vi "Begin.vi"() -> (0 "CameraDevRef 2":T1, 1 "CameraDevRef":T1)   [LabVIEW 2011]
doc: "Called before other user functions, this VI is expected to open initial I/O refnums, load in file data, and do all program initialization. Notice that the <B>error out</B> terminal is simply used for data flow. Wiring it to other structures or subVIs ensures that this VI runs first."
uses:
  <vilib>/Rock Robotics/WPI/Camera/WPI_CameraDevRef.ctl
  <vilib>/Rock Robotics/SystemInterfaces/DIO/FPGA_DIOPWMChannel.ctl
  <vilib>/Rock Robotics/WPI/Joystick/WPI_JoystickDeviceEnum.ctl
  <vilib>/Rock Robotics/SystemInterfaces/AI/FPGA_AIChannel.ctl
  <vilib>/Rock Robotics/SystemInterfaces/DIO/FPGA_DIORelayChannel.ctl
  <vilib>/Rock Robotics/SystemInterfaces/DIO/FPGA_DIOChannel.ctl
  <vilib>/Rock Robotics/SystemInterfaces/AI/FPGA_AIGyroChannel.ctl
  <vilib>/Rock Robotics/WPI/Relay/WPI_RelayDirection.ctl
  <vilib>/Rock Robotics/WPI/Encoder/WPI_EncoderType.ctl
  <vilib>/Rock Robotics/WPI/DriverStation/DriverStationLCD/WPI_DriverStationLCDLCDLine.ctl
  <vilib>/Rock Robotics/WPI/MotorControl/WPI_MotorControlOpen Victor.vi
  <vilib>/Rock Robotics/WPI/MotorControl/WPI_MotorControlOpen Jaguar.vi
  Robot Global Data.vi
  <vilib>/Utility/file.llb/Read From Spreadsheet File (DBL).vi
  <vilib>/Rock Robotics/WPI/Counter/WPI_CounterDigitalInputToDigitalSource.vi
  <vilib>/Rock Robotics/SystemInterfaces/Typedef/FPGA_TypedefDigitalModule.ctl
  <vilib>/Rock Robotics/SystemInterfaces/Typedef/FPGA_TypedefAnalogModule.ctl
panel:
  in  "Default Shooter in Feet":i32=13
  out "Path and file":string
  in  "Balls In Robot At Start":dbl=2.0
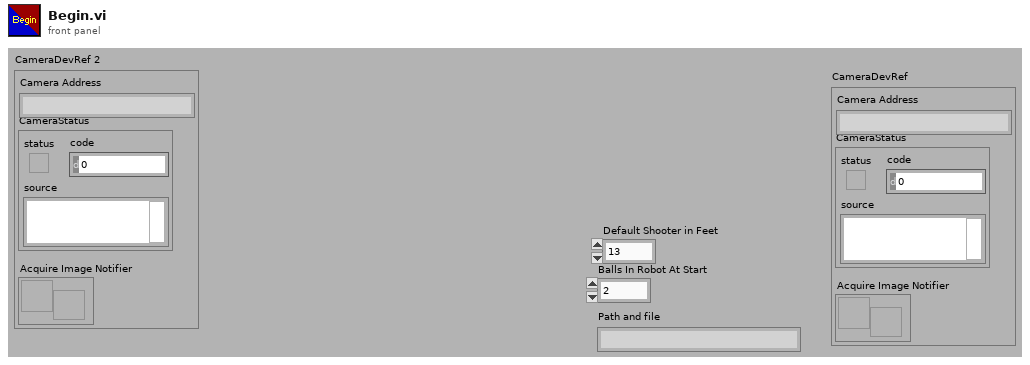
[diagram p1: front panel]
types:
  T1 = typedef "WPI_CameraDevRef.ctl" = cluster{"Camera Address":string, "CameraStatus":errorcluster, "Acquire Image Notifier":refnum<notifier>}
  T2 = typedef "FPGA_DIOChannel.ctl" = enum8{"DIO 1", "DIO 2", "DIO 3", "DIO 4", "DIO 5", "DIO 6", "DIO 7", "DIO 8", "DIO 9", "DIO 10", "DIO 11", "DIO 12", "DIO 13", "DIO 14", "Invalid"}
  T3 = typedef "FPGA_DIOPWMChannel.ctl" = enum8{"PWM 1", "PWM 2", "PWM 3", "PWM 4", "PWM 5", "PWM 6", "PWM 7", "PWM 8", "PWM 9", "PWM 10", "Invalid"}
  T4 = typedef "WPI_DriverStationLCDLCDLine.ctl" = enum16{"Main - Line 1", "User - Line 2", "User - Line 3", "User - Line 4", "User - Line 5", "User - Line 6"}
  T5 = typedef "WPI_EncoderType.ctl" = enum16{"1x", "2x", "4x"}
  T6 = typedef "FPGA_DIORelayChannel.ctl" = enum8{"Relay 1", "Relay 2", "Relay 3", "Relay 4", "Relay 5", "Relay 6", "Relay 7", "Relay 8", "Invalid"}
  T7 = typedef "WPI_RelayDirection.ctl" = enum16{"Both directions", "Forward only", "Reverse only"}
  T8 = typedef "FPGA_AIGyroChannel.ctl" = enum8{"AI 1", "AI 2", "Invalid"}
  T9 = typedef "FPGA_AIChannel.ctl" = enum8{"AI 1", "AI 2", "AI 3", "AI 4", "AI 5", "AI 6", "AI 7", "AI 8", "Invalid"}
  T10 = typedef "WPI_JoystickDeviceEnum.ctl" = enum16{"USB 1", "USB 2", "USB 3", "USB 4", "Kinect 1", "Kinect 2"}
  T11 = typedef "WPI_CameraImageSize.ctl" = enum16{"640x480", "320x240", "160x120"}
  T12 = cluster{"fps":i32, "compression":i32, "Image Size":T11}
  T13 = typedef "WPI_MotorControlDeviceRef.ctl" = cluster{"DeviceStatus":errorcluster, "Type":enum16{"PWM", "CAN"}, "PWM":cluster{"Digital Module":T14, "PWM Channel":T3, "DeadBand":T15}, "CAN":cluster{"Device Number":u8, "Control Mode":T16, "Semaphore":T17, "Max Vout":dbl}, "Invert":bool, "TransformRef":T18, "InvTransformRef":T18}
  T14 = typedef "FPGA_TypedefDigitalModule.ctl" = enum16{"Digital Module 1", "Digital Module 2"}
  T15 = typedef "WPI_PWMDeadband.ctl" = cluster{"Name":string, "maxPositivePwm":i32, "minPositivePwm":i32, "centerPwm":i32, "maxNegativePwm":i32, "minNegativePwm":i32, "angularRange":u16}
  T16 = typedef "WPI_CANJaguar_ControlMode.ctl" = enum8{"Percent VBus", "Current", "Speed", "Position", "Voltage"}
  T17 = typedef "Semaphore RefNum" = refnum<k1>
  T18 = typedef "WPI_PWMTransform_ConPane.ctl" = refnum<vi>
  T19 = typedef "WPI_ServoDeviceRef.ctl" = cluster{"DeviceStatus":errorcluster, "Digital Module":T14, "PWM Channel":T3, "DeadBand":T15}
  T20 = typedef "WPI_AnalogChannelDevRef.ctl" = cluster{"DevStatus":errorcluster, "Analog Module":T21, "Analog Channel":T9}
  T21 = typedef "FPGA_TypedefAnalogModule.ctl" = enum16{"Analog Module 1", "Analog Module 2"}
  T22 = typedef "WPI_CameraWhite Balance Values.ctl" = enum16{"Auto", "Fixed indoor", "Fixed outdoor 1", "Fixed outdoor 2", "Fixed fluorescent 1", "Fixed fluorescent 2", "Hold current"}
  T23 = typedef "WPI_JoystickDevRef.ctl" = cluster{"Device":T10}
  T24 = typedef "WPI_RelayDevRef.ctl" = cluster{"DevStatus":errorcluster, "Relay Channel":T6, "Digital Module":T14, "Relay Direction":T7}
  T25 = typedef "WPI_CameraExposure Values.ctl" = enum16{"Auto", "Flicker-free 50 Hz", "Flicker-free 60 Hz", "Hold current"}
  T26 = typedef "WPI_DigitalInputDevRef.ctl" = cluster{"DevStatus":errorcluster, "DIO Channel":T2, "Digital Module":T14}
  T27 = typedef "FPGA_CounterEncoderSourceConvertionLVSourceType.ctl" = cluster{"DevStatus":errorcluster, "AnalogTriggerMode?":bool, "DigitalMode":cluster{"Digital Module":T14, "DIO Channel":T28}, "AnalogTriggerMode":cluster{"AnalogTriggerIndex":T29, "OutputType":T30}}
  T28 = typedef "FPGA_DIODigitalSourceChannel.ctl" = enum8{"DIO 1", "DIO 2", "DIO 3", "DIO 4", "DIO 5", "DIO 6", "DIO 7", "DIO 8", "DIO 9", "DIO 10", "DIO 11", "DIO 12", "DIO 13", "DIO 14", "Disabled"}
  T29 = typedef "FPGA_AnalogTriggerIndex.ctl" = enum8{"Trig 0", "Trig 1", "Trig 2", "Trig 3", "Trig 4", "Trig 5", "Trig 6", "Trig 7", "Invalid"}
  T30 = typedef "FPGA_AnalogTriggerOutType.ctl" = enum16{"InWindow", "TriggerState", "Rising", "Falling"}
  T31 = typedef "WPI_EncoderDevRef.ctl" = cluster{"DevStatus":errorcluster, "EncoderIndex":T32, "CounterIndex":T33, "DistancePerCount":dbl, "Decoding Type":T5}
  T32 = typedef "FPGA_EncoderIdx.ctl" = enum8{"Enc 0", "Enc 1", "Enc 2", "Enc 3", "Invalid"}
  T33 = typedef "FPGA_CounterCtrSystemIndex.ctl" = enum8{"Ctr 0", "Ctr 1", "Ctr 2", "Ctr 3", "Ctr 4", "Ctr 5", "Ctr 6", "Ctr 7", "Invalid"}
  T34 = typedef "WPI_GyroDevRef.ctl" = cluster{"DevStatus":errorcluster, "Analog Module":T21, "Analog Channel":T9, "Offset":dbl, "Gain (VoltsPerDegree/Second)":dbl}
  T35 = typedef "WPI_UltrasonicDeviceRef.ctl" = cluster{"DevStatus":errorcluster, "Ping Digital Module":T14, "Echo Digital Module":T14, "Ping Channel":T2, "Echo Channel":T2, "CntIndex":T33}
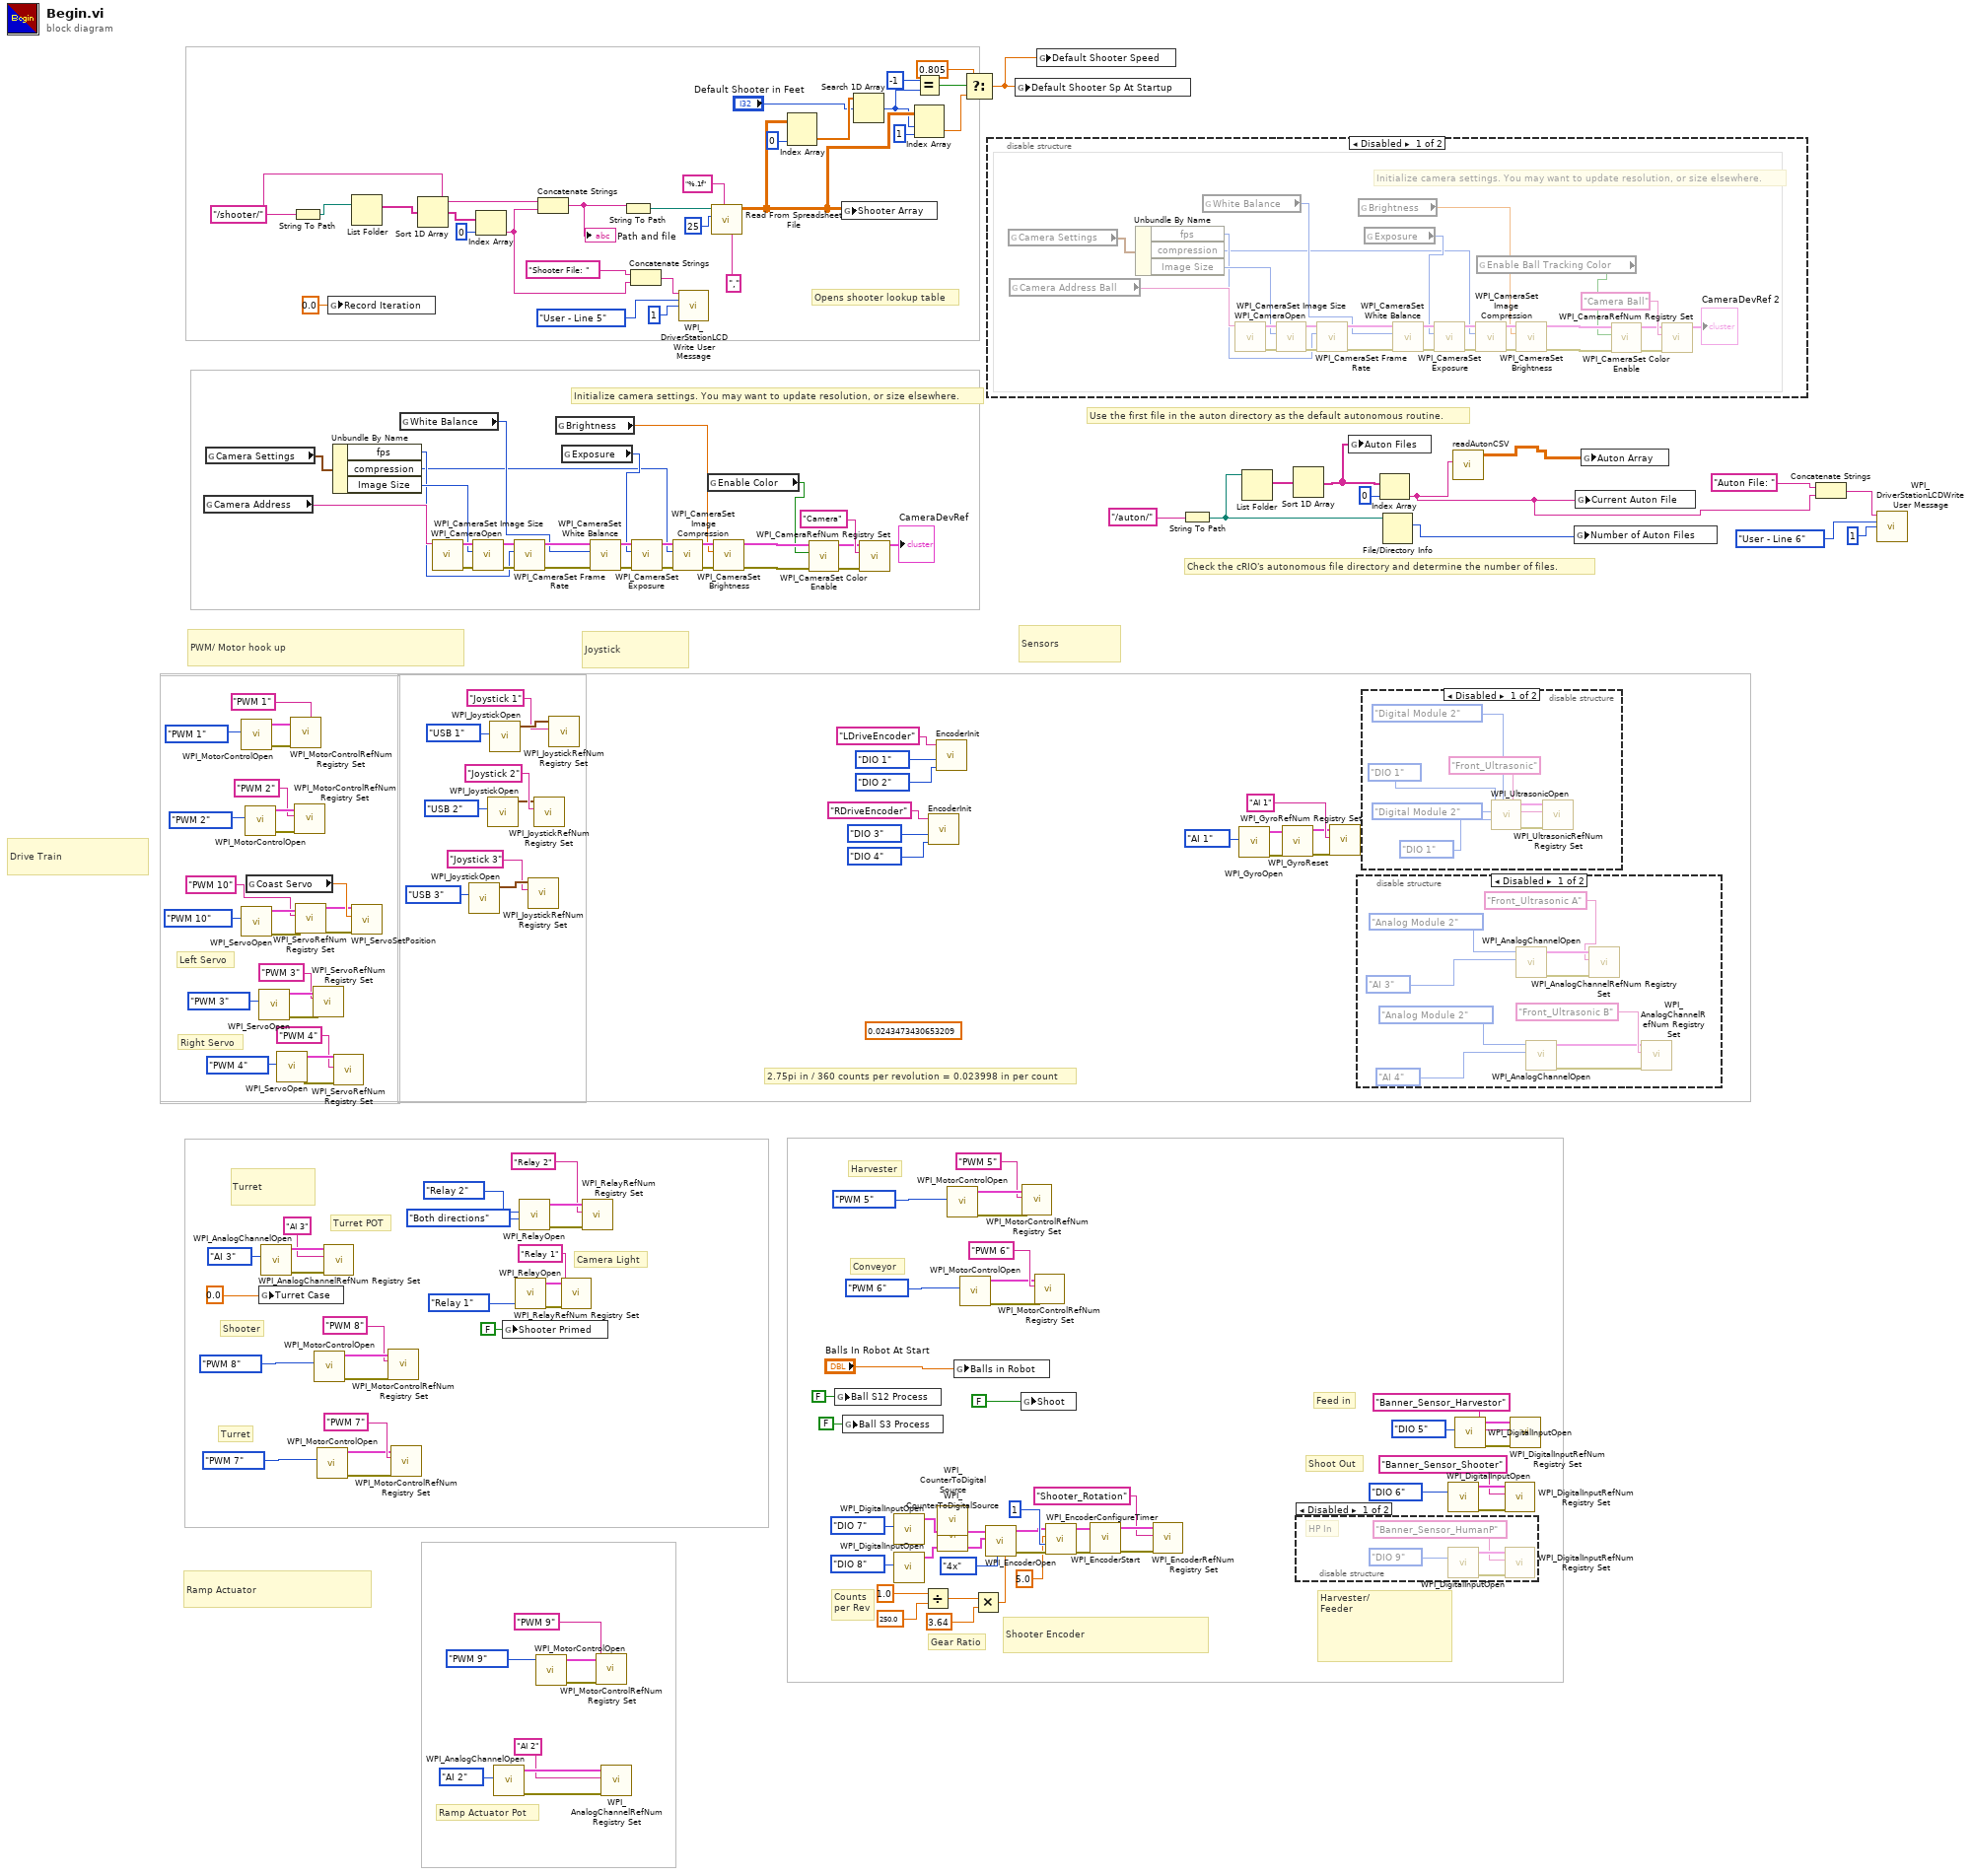
[diagram p0: block diagram]
diagram:
  (unwired) 0.0243473430653209 ("DistancePerCount")
  w70 = "/shooter/" ("string")
  # "Shooter Encoder"
  # "Counts\nper Rev"
  # "Gear Ratio"
  # "Check the cRIO's autonomous file directory and determine the number of files."
  # "Use the first file in the auton directory as the default autonomous routine."
  # "2.75pi in / 360 counts per revolution = 0.023998 in per count"
  # "Opens shooter lookup table"
  # "Shoot Out"
  # "Feed in"
  # "Harvester"
  # "Conveyor"
  # "Shooter"
  # "Initialize camera settings. You may want to update resolution, or size elsewhere."
  # "Camera Light"
  # "Ramp Actuator Pot"
  # "Turret POT"
  # "Turret"
  # "Right Servo"
  # "Left Servo"
  # "Harvester/\nFeeder"
  # "Turret"
  # "Ramp Actuator"
  # "Drive Train"
  # "Sensors"
  # "Joystick"
  # "PWM/ Motor hook up"
  n1 = global read "Robot Global Data.vi" "Camera Address"() -> (w123:string)
  n2 = global read "Robot Global Data.vi" "Camera Settings"() -> (w122:T12)
  n3 = call-poly <vilib>:"WPI_MotorControlOpen.vi"("PWM Channel"=FPGA_DIOPWMChannel."PWM 1") -> ("error out"=w163:errorcluster, "MotorControlDeviceRef"=w165:T13)  [unwired: 9 in]
  n4 = call <vilib>:"WPI_ServoOpen.vi"("PWM Channel"=FPGA_DIOPWMChannel."PWM 10") -> ("error out"=w19:errorcluster, "ServoDeviceRef"=w23:T19)  [unwired: 9 in]
  n5 = call-poly <vilib>:"WPI_MotorControlOpen.vi"("PWM Channel"=FPGA_DIOPWMChannel."PWM 2") -> ("error out"=w161:errorcluster, "MotorControlDeviceRef"=w159:T13)  [unwired: 9 in]
  n6 = global read "Robot Global Data.vi" "Coast Servo"() -> (w24:dbl)
  n7 = call <vilib>:"WPI_ServoOpen.vi"("PWM Channel"=FPGA_DIOPWMChannel."PWM 3") -> ("error out"=w176:errorcluster, "ServoDeviceRef"=w181:T19)  [unwired: 9 in]
  n8 = global write "Robot Global Data.vi" "Turret Case"(0.0 ("Return To Home Case")) -> ()
  n9 = call <vilib>:"WPI_AnalogChannelOpen.vi"("Analog Channel"=FPGA_AIChannel."AI 3") -> ("error out"=w152:errorcluster, "AIDeviceRef"=w153:T20)  [unwired: 9 in]
  n10 = call <vilib>:"WPI_ServoOpen.vi"("PWM Channel"=FPGA_DIOPWMChannel."PWM 4") -> ("error out"=w175:errorcluster, "ServoDeviceRef"=w179:T19)  [unwired: 9 in]
  n11 = call <vilib>:"WPI_MotorControlRefNum Registry Set.vi"("error in (no error)"=w163, "refnum name"="PWM 1", "MotorControlDevRef"=w165) -> ()  [unwired: 7 in, 2 out]
  n12 = String To Path(string=w70) -> (path=w79:path)
  n13 = call <vilib>:"WPI_MotorControlRefNum Registry Set.vi"("error in (no error)"=w161, "refnum name"="PWM 2", "MotorControlDevRef"=w159) -> ()  [unwired: 7 in, 2 out]
  n14 = call <vilib>:"WPI_ServoRefNum Registry Set.vi"("error in (no error)"=w19, "refnum name"="PWM 10", "ServoDeviceRef"=w23) -> ("error out"=w20:errorcluster, "ServoDeviceRef"=w21:T19)  [unwired: 7 in]
  n15 = call <vilib>:"WPI_ServoRefNum Registry Set.vi"("error in (no error)"=w176, "refnum name"="PWM 3", "ServoDeviceRef"=w181) -> ()  [unwired: 7 in, 2 out]
  n16 = call-poly <vilib>:"WPI_MotorControlOpen.vi"("PWM Channel"=FPGA_DIOPWMChannel."PWM 8") -> ("error out"=w106:errorcluster, "MotorControlDeviceRef"=w108:T13)  [unwired: 9 in]
  n17 = call-poly <vilib>:"WPI_MotorControlOpen.vi"("PWM Channel"=FPGA_DIOPWMChannel."PWM 7") -> ("error out"=w157:errorcluster, "MotorControlDeviceRef"=w155:T13)  [unwired: 9 in]
  n18 = call <vilib>:"WPI_AnalogChannelRefNum Registry Set.vi"("error in (no error)"=w152, "refnum name"="AI 3", "AIDeviceRef"=w153) -> ()  [unwired: 7 in, 2 out]
  n19 = global write "Robot Global Data.vi" "Record Iteration"(0.0 ("Record Iteration")) -> ()
  n20 = Unbundle By Name(w122) -> ("fps"=w120:i32, "compression"=w117:i32, "Image Size"=w121:T11)
  n21 = call <vilib>:"WPI_ServoRefNum Registry Set.vi"("error in (no error)"=w175, "refnum name"="PWM 4", "ServoDeviceRef"=w179) -> ()  [unwired: 7 in, 2 out]
  n22 = List Folder(path=w79) -> (filenames=w78:string[])  [unwired: 1 in, 5 out]
  n23 = call <vilib>:"WPI_ServoSetPosition.vi"("error in (no error)"=w20, "Position"=w24, "ServoDeviceRef"=w21) -> ()  [unwired: 7 in, 2 out]
  n24 = call <vilib>:"WPI_MotorControlRefNum Registry Set.vi"("error in (no error)"=w106, "refnum name"="PWM 8", "MotorControlDevRef"=w108) -> ()  [unwired: 7 in, 2 out]
  n25 = call <vilib>:"WPI_MotorControlRefNum Registry Set.vi"("error in (no error)"=w157, "refnum name"="PWM 7", "MotorControlDevRef"=w155) -> ()  [unwired: 7 in, 2 out]
  n26 = global read "Robot Global Data.vi" "White Balance"() -> (w119:T22)
  n27 = Sort 1D Array(array=w78) -> (sorted array=w77:string[])
  n28 = call <vilib>:"WPI_CameraOpen.vi"("Camera Address"=w123) -> ("error out"=w129:errorcluster, "CameraDevRef"=w130:T1)  [unwired: 1 in, 8 out]
  n29 = call <vilib>:"WPI_JoystickOpen.vi"("JoystickDevice"=WPI_JoystickDeviceEnum."USB 3") -> ("JoystickDevRef"=w168:T23)  [unwired: 10 in]
  n30 = call <vilib>:"WPI_CameraSet Image Size.vi"("error in (no error)"=w129, "Image Size"=w121, "CameraDevRef"=w130) -> ("error out"=w128:errorcluster, "CameraDevRef Out"=w131:T1)  [unwired: 7 out]
  n31 = Index Array(array=w77, index=0) -> (element=w30:string)
  n32 = call <vilib>:"WPI_JoystickOpen.vi"("JoystickDevice"=WPI_JoystickDeviceEnum."USB 2") -> ("JoystickDevRef"=w171:T23)  [unwired: 10 in]
  n33 = call <vilib>:"WPI_JoystickOpen.vi"("JoystickDevice"=WPI_JoystickDeviceEnum."USB 1") -> ("JoystickDevRef"=w174:T23)  [unwired: 10 in]
  n34 = call <vilib>:"WPI_AnalogChannelOpen.vi"("Analog Channel"=FPGA_AIChannel."AI 2") -> ("error out"=w147:errorcluster, "AIDeviceRef"=w148:T20)  [unwired: 9 in]
  n35 = global write "Robot Global Data.vi" "Shooter Primed"(FALSE ("Ball S3 Process")) -> ()
  n36 = call <vilib>:"WPI_CameraSet Frame Rate.vi"("error in (no error)"=w128, "Frame Rate (fps)"=w120, "CameraDevRef"=w131) -> ("error out"=w127:errorcluster, "CameraDevRef Out"=w133:T1)  [unwired: 7 out]
  n37 = call <vilib>:"WPI_RelayOpen.vi"("Relay Channel"=FPGA_DIORelayChannel."Relay 1") -> ("error out"=w140:errorcluster, "RelayDevRef"=w139:T24)  [unwired: 9 in]
  n38 = call <vilib>:"WPI_RelayOpen.vi"("Relay Direction"=WPI_RelayDirection."Both directions", "Relay Channel"=FPGA_DIORelayChannel."Relay 2") -> ("error out"=w66:errorcluster, "RelayDevRef"=w67:T24)  [unwired: 8 in]
  n39 = call <vilib>:"WPI_JoystickRefNum Registry Set.vi"("refnum name"="Joystick 3", "JoystickDevRef"=w168) -> ()  [unwired: 8 in, 2 out]
  n40 = call <vilib>:"WPI_JoystickRefNum Registry Set.vi"("refnum name"="Joystick 2", "JoystickDevRef"=w171) -> ()  [unwired: 8 in, 2 out]
  n41 = call-poly <vilib>:"WPI_MotorControlOpen.vi"("PWM Channel"=FPGA_DIOPWMChannel."PWM 9") -> ("error out"=w143:errorcluster, "MotorControlDeviceRef"=w144:T13)  [unwired: 9 in]
  n42 = Concatenate Strings(w70, w30) -> (w72:string)
  "Path and file" <- w72
  n43 = call <vilib>:"WPI_JoystickRefNum Registry Set.vi"("refnum name"="Joystick 1", "JoystickDevRef"=w174) -> ()  [unwired: 8 in, 2 out]
  n44 = global read "Robot Global Data.vi" "Brightness"() -> (w116:dbl)
  n45 = global read "Robot Global Data.vi" "Exposure"() -> (w118:T25)
  n46 = call <vilib>:"WPI_RelayRefNum Registry Set.vi"("error in (no error)"=w140, "refnum name"="Relay 1", "RelayDevRef"=w139) -> ()  [unwired: 7 in, 2 out]
  n47 = call <vilib>:"WPI_RelayRefNum Registry Set.vi"("error in (no error)"=w66, "refnum name"="Relay 2", "RelayDevRef"=w67) -> ()  [unwired: 7 in, 2 out]
  n48 = call <vilib>:"WPI_CameraSet White Balance.vi"("error in (no error)"=w127, "White Balance"=w119, "CameraDevRef"=w133) -> ("error out"=w126:errorcluster, "CameraDevRef Out"=w132:T1)  [unwired: 7 out]
  n49 = call <vilib>:"WPI_MotorControlRefNum Registry Set.vi"("error in (no error)"=w143, "refnum name"="PWM 9", "MotorControlDevRef"=w144) -> ()  [unwired: 7 in, 2 out]
  n50 = call <vilib>:"WPI_AnalogChannelRefNum Registry Set.vi"("error in (no error)"=w147, "refnum name"="AI 2", "AIDeviceRef"=w148) -> ()  [unwired: 7 in, 2 out]
  n51 = String To Path(string=w72) -> (path=w71:path)
  n52 = Concatenate Strings("Shooter File: ", w30) -> (w28:string)
  n53 = call <vilib>:"WPI_CameraSet Exposure.vi"("error in (no error)"=w126, "Exposure"=w118, "CameraDevRef"=w132) -> ("error out"=w125:errorcluster, "CameraDevRef Out"=w135:T1)  [unwired: 7 out]
  n54 = call <vilib>:"WPI_CameraSet Image Compression.vi"("error in (no error)"=w125, "Compression"=w117, "CameraDevRef"=w135) -> ("error out"=w124:errorcluster, "CameraDevRef Out"=w134:T1)  [unwired: 7 out]
  n55 = call <vilib>:"WPI_DriverStationLCDWrite User Message.vi"("line text"=w28, "line"=WPI_DriverStationLCDLCDLine."User - Line 5", "starting column"=i8 1) -> ()  [unwired: 2 in, 11 out]
  n56 = global read "Robot Global Data.vi" "Enable Color"() -> (w111:bool)
  n57 = call-poly <vilib>:"Read From Spreadsheet File.vi"("delimiter (\\t)"="," ("delimiter (\\t)"), "format (%.3f)"="%.1f", "number of rows (all:-1)"=25, "file path (dialog if empty)"=w71) -> ("all rows"=w14:dbl[][])  [unwired: 1 in, 6 out]
  n58 = call <vilib>:"WPI_CameraSet Brightness.vi"("error in (no error)"=w124, "Brightness"=w116, "CameraDevRef"=w134) -> ("error out"=w114:errorcluster, "CameraDevRef Out"=w115:T1)  [unwired: 7 out]
  n59 = Index Array(array=w14, index (col)=0 ("disabled index (col)")) -> (element=w16:dbl[])  [unwired: 1 in]
  n60 = call <vilib>:"WPI_CameraSet Color Enable.vi"("error in (no error)"=w114, "Color Enabled"=w111, "CameraDevRef"=w115) -> ("error out"=w112:errorcluster, "CameraDevRef Out"=w113:T1)  [unwired: 7 in]
  n61 = global write "Robot Global Data.vi" "Ball S12 Process"(FALSE ("Ball S12 Process")) -> ()
  n62 = global write "Robot Global Data.vi" "Shooter Array"(w14) -> ()
  n63 = global write "Robot Global Data.vi" "Ball S3 Process"(FALSE ("Ball S3 Process")) -> ()
  n64 = Search 1D Array(1D array=w16, element="Default Shooter in Feet") -> (index of element=w13:i32)  [unwired: 1 in]
  n65 = call <vilib>:"WPI_CameraRefNum Registry Set.vi"("error in (no error)"=w112, "refnum name"="Camera", "CameraDevRef"=w113) -> ("CameraDevRef"=→"CameraDevRef":T1)  [unwired: 8 out]
  n66 = call <vilib>:"WPI_DigitalInputOpen.vi"("DIO Channel"=FPGA_DIOChannel."DIO 7") -> ("DigitalInputDevRef"=w40:T26)  [unwired: 9 in, 1 out]
  n67 = call <vilib>:"WPI_DigitalInputOpen.vi"("DIO Channel"=FPGA_DIOChannel."DIO 8") -> ("DigitalInputDevRef"=w43:T26)  [unwired: 9 in, 1 out]
  n68 = Equal?(x=-1, y=w13) -> (x = y?=w11:bool)
  n69 = Index Array(array=w14, index (row)=w13, index (col)=1) -> (element=w9:dbl)
  n70 = Divide(x=1.0, y=250.0) -> (x/y=w37:dbl)
  n71 = call "EncoderInit.vi"("refnum name"="RDriveEncoder", "DIO Channel"=FPGA_DIOChannel."DIO 3", "DIO Channel 2"=FPGA_DIOChannel."DIO 4" ("DIO Channel")) -> ()  [unwired: 8 in]
  n72 = call "EncoderInit.vi"("refnum name"="LDriveEncoder", "DIO Channel"=FPGA_DIOChannel."DIO 1", "DIO Channel 2"=FPGA_DIOChannel."DIO 2" ("DIO Channel")) -> ()  [unwired: 8 in]
  n73 = call-poly <vilib>:"WPI_CounterToDigitalSource.vi"("DigitalInputDevRef"=w40) -> ("Digital Source"=w39:T27)  [unwired: 6 in]
  n74 = call-poly <vilib>:"WPI_CounterToDigitalSource.vi"("DigitalInputDevRef"=w43) -> ("Digital Source"=w44:T27)  [unwired: 6 in]
  n75 = call-poly <vilib>:"WPI_MotorControlOpen.vi"("PWM Channel"=FPGA_DIOPWMChannel."PWM 5") -> ("error out"=w102:errorcluster, "MotorControlDeviceRef"=w104:T13)  [unwired: 9 in]
  n76 = global write "Robot Global Data.vi" "Balls in Robot"("Balls In Robot At Start") -> ()
  n77 = call-poly <vilib>:"WPI_MotorControlOpen.vi"("PWM Channel"=FPGA_DIOPWMChannel."PWM 6") -> ("error out"=w101:errorcluster, "MotorControlDeviceRef"=w99:T13)  [unwired: 9 in]
  n78 = Select(t=0.805, s=w11, f=w9) -> (s? t:f=w7:dbl)
  n79 = Multiply(x=w37, y=3.64) -> (x*y=w35:dbl)
  n80 = call <vilib>:"WPI_EncoderOpen.vi"("DistancePerCount"=w35, "Decoding Type"=WPI_EncoderType."4x", "BSource"=w44, "ASource"=w39) -> ("error out"=w47:errorcluster, "EncoderDevRef"=w48:T31)  [unwired: 6 in]
  n81 = disable-structure shown="Disabled" {
    frame Disabled {
      # "Initialize camera settings. You may want to update resolution, or size elsewhere."
      n82 = global read "Robot Global Data.vi" "Camera Settings"() -> (w195:T12)
      n83 = global read "Robot Global Data.vi" "Camera Address Ball"() -> (w196:string)
      n84 = Unbundle By Name(w195) -> ("fps"=w193:i32, "compression"=w190:i32, "Image Size"=w194:T11)
      n85 = global read "Robot Global Data.vi" "White Balance"() -> (w192:T22)
      n86 = call <vilib>:"WPI_CameraOpen.vi"("Camera Address"=w196) -> ("error out"=w202:errorcluster, "CameraDevRef"=w203:T1)  [unwired: 1 in, 8 out]
      n87 = call <vilib>:"WPI_CameraSet Image Size.vi"("error in (no error)"=w202, "Image Size"=w194, "CameraDevRef"=w203) -> ("error out"=w201:errorcluster, "CameraDevRef Out"=w204:T1)  [unwired: 7 out]
      n88 = call <vilib>:"WPI_CameraSet Frame Rate.vi"("error in (no error)"=w201, "Frame Rate (fps)"=w193, "CameraDevRef"=w204) -> ("error out"=w200:errorcluster, "CameraDevRef Out"=w206:T1)  [unwired: 7 out]
      n89 = global read "Robot Global Data.vi" "Brightness"() -> (w189:dbl)
      n90 = global read "Robot Global Data.vi" "Exposure"() -> (w191:T25)
      n91 = call <vilib>:"WPI_CameraSet White Balance.vi"("error in (no error)"=w200, "White Balance"=w192, "CameraDevRef"=w206) -> ("error out"=w199:errorcluster, "CameraDevRef Out"=w205:T1)  [unwired: 7 out]
      n92 = call <vilib>:"WPI_CameraSet Exposure.vi"("error in (no error)"=w199, "Exposure"=w191, "CameraDevRef"=w205) -> ("error out"=w198:errorcluster, "CameraDevRef Out"=w208:T1)  [unwired: 7 out]
      n93 = call <vilib>:"WPI_CameraSet Image Compression.vi"("error in (no error)"=w198, "Compression"=w190, "CameraDevRef"=w208) -> ("error out"=w197:errorcluster, "CameraDevRef Out"=w207:T1)  [unwired: 7 out]
      n94 = global read "Robot Global Data.vi" "Enable Ball Tracking Color"() -> (w184:bool)
      n95 = call <vilib>:"WPI_CameraSet Brightness.vi"("error in (no error)"=w197, "Brightness"=w189, "CameraDevRef"=w207) -> ("error out"=w187:errorcluster, "CameraDevRef Out"=w188:T1)  [unwired: 7 out]
      n96 = call <vilib>:"WPI_CameraSet Color Enable.vi"("error in (no error)"=w187, "Color Enabled"=w184, "CameraDevRef"=w188) -> ("error out"=w185:errorcluster, "CameraDevRef Out"=w186:T1)  [unwired: 7 in]
      n97 = call <vilib>:"WPI_CameraRefNum Registry Set.vi"("error in (no error)"=w185, "refnum name"="Camera Ball", "CameraDevRef"=w186) -> ("CameraDevRef"=→"CameraDevRef 2":T1)  [unwired: 8 out]
    }
    frame Enabled {
    }
  }
  n98 = global write "Robot Global Data.vi" "Default Shooter Sp At Startup"(w7) -> ()
  n99 = global write "Robot Global Data.vi" "Shoot"(FALSE ("Ball S12 Process")) -> ()
  n100 = call <vilib>:"WPI_MotorControlRefNum Registry Set.vi"("error in (no error)"=w102, "refnum name"="PWM 5", "MotorControlDevRef"=w104) -> ()  [unwired: 7 in, 2 out]
  n101 = call <vilib>:"WPI_MotorControlRefNum Registry Set.vi"("error in (no error)"=w101, "refnum name"="PWM 6", "MotorControlDevRef"=w99) -> ()  [unwired: 7 in, 2 out]
  n102 = global write "Robot Global Data.vi" "Default Shooter Speed"(w7) -> ()
  n103 = call <vilib>:"WPI_EncoderConfigureTimer.vi"("error in (no error)"=w47, "Number Samples to Average"=u8 1, "Minimum Rate"=5.0, "EncoderDevRef"=w48) -> ("error out"=w51:errorcluster, "EncoderDevRef"=w50:T31)  [unwired: 6 in]
  n104 = call <vilib>:"WPI_EncoderStart.vi"("error in (no error)"=w51, "EncoderDevRef"=w50) -> ("error out"=w53:errorcluster, "EncoderDevRef"=w52:T31)  [unwired: 8 in]
  n105 = call <vilib>:"WPI_EncoderRefNum Registry Set.vi"("error in (no error)"=w53, "refnum name"="Shooter_Rotation", "EncoderDevRef"=w52) -> ()  [unwired: 7 in, 2 out]
  n106 = String To Path(string="/auton/") -> (path=w60:path)
  n107 = call <vilib>:"WPI_GyroOpen.vi"("Analog Channel"=FPGA_AIGyroChannel."AI 1") -> ("error out"=w82:errorcluster, "GyroDevRef"=w83:T34)  [unwired: 8 in, 1 out]
  n108 = List Folder(path=w60) -> (filenames=w59:string[])  [unwired: 1 in, 5 out]
  n109 = call <vilib>:"WPI_GyroReset.vi"("error in (no error)"=w82, "GyroDevRef"=w83) -> ("error out"=w81:errorcluster, "GyroDevRef"=w80:T34)  [unwired: 8 in]
  n110 = Sort 1D Array(array=w59) -> (sorted array=w57:string[])
  n111 = disable-structure shown="Disabled" {
    frame Disabled {
      # "HP In"
      n112 = call <vilib>:"WPI_DigitalInputOpen.vi"("DIO Channel"=FPGA_DIOChannel."DIO 9") -> ("error out"=w212:errorcluster, "DigitalInputDevRef"=w211:T26)  [unwired: 9 in]
      n113 = call <vilib>:"WPI_DigitalInputRefNum Registry Set.vi"("error in (no error)"=w212, "refnum name"="Banner_Sensor_HumanP", "DigitalInputDevRef"=w211) -> ()  [unwired: 7 in, 2 out]
    }
    frame Enabled {
    }
  }
  n114 = call <vilib>:"WPI_GyroRefNum Registry Set.vi"("error in (no error)"=w81, "refnum name"="AI 1", "GyroDevRef"=w80) -> ()  [unwired: 7 in, 2 out]
  n115 = global write "Robot Global Data.vi" "Auton Files"(w57) -> ()
  n116 = disable-structure shown="Disabled" {
    frame Disabled {
      n117 = call <vilib>:"WPI_AnalogChannelOpen.vi"("Analog Channel"=FPGA_AIChannel."AI 3", "Analog Module (Module 1)"=FPGA_TypedefAnalogModule."Analog Module 2") -> ("error out"=w219:errorcluster, "AIDeviceRef"=w218:T20)  [unwired: 8 in]
      n118 = call <vilib>:"WPI_AnalogChannelOpen.vi"("Analog Channel"=FPGA_AIChannel."AI 4", "Analog Module (Module 1)"=FPGA_TypedefAnalogModule."Analog Module 2") -> ("error out"=w214:errorcluster, "AIDeviceRef"=w215:T20)  [unwired: 8 in]
      n119 = call <vilib>:"WPI_AnalogChannelRefNum Registry Set.vi"("error in (no error)"=w219, "refnum name"="Front_Ultrasonic A", "AIDeviceRef"=w218) -> ()  [unwired: 7 in, 2 out]
      n120 = call <vilib>:"WPI_AnalogChannelRefNum Registry Set.vi"("error in (no error)"=w214, "refnum name"="Front_Ultrasonic B", "AIDeviceRef"=w215) -> ()  [unwired: 7 in, 2 out]
    }
    frame Enabled {
    }
  }
  n121 = disable-structure shown="Disabled" {
    frame Disabled {
      n122 = call <vilib>:"WPI_UltrasonicOpen.vi"("Ping Digital Module (Module 1)"=FPGA_TypedefDigitalModule."Digital Module 2", "Echo DIO Channel"=FPGA_DIOChannel."DIO 1", "Echo Digital Module (Module 1)"=FPGA_TypedefDigitalModule."Digital Module 2", "Ping DIO Channel"=FPGA_DIOChannel."DIO 1") -> ("error out"=w230:errorcluster, "UltrasonicDevRef"=w229:T35)  [unwired: 6 in]
      n123 = call <vilib>:"WPI_UltrasonicRefNum Registry Set.vi"("error in (no error)"=w230, "refnum name"="Front_Ultrasonic", "UltrasonicDevRef"=w229) -> ()  [unwired: 7 in, 2 out]
    }
    frame Enabled {
    }
  }
  n124 = Index Array(array=w57, index=0) -> (element=w26:string)
  n125 = File/Directory Info(path=w60) -> (size=w62:i64)  [unwired: 1 in, 6 out]
  n126 = call <vilib>:"WPI_DigitalInputOpen.vi"("DIO Channel"=FPGA_DIOChannel."DIO 6") -> ("error out"=w92:errorcluster, "DigitalInputDevRef"=w91:T26)  [unwired: 9 in]
  n127 = call "readAutonCSV.vi"("AutonFile"=w26) -> ("AutonArray"=w56:dbl[][])  [unwired: 7 in]
  n128 = call <vilib>:"WPI_DigitalInputOpen.vi"("DIO Channel"=FPGA_DIOChannel."DIO 5") -> ("error out"=w95:errorcluster, "DigitalInputDevRef"=w94:T26)  [unwired: 9 in]
  n129 = call <vilib>:"WPI_DigitalInputRefNum Registry Set.vi"("error in (no error)"=w92, "refnum name"="Banner_Sensor_Shooter", "DigitalInputDevRef"=w91) -> ()  [unwired: 7 in, 2 out]
  n130 = call <vilib>:"WPI_DigitalInputRefNum Registry Set.vi"("error in (no error)"=w95, "refnum name"="Banner_Sensor_Harvestor", "DigitalInputDevRef"=w94) -> ()  [unwired: 7 in, 2 out]
  n131 = global write "Robot Global Data.vi" "Number of Auton Files"(w62) -> ()
  n132 = global write "Robot Global Data.vi" "Current Auton File"(w26) -> ()
  n133 = global write "Robot Global Data.vi" "Auton Array"(w56) -> ()
  n134 = Concatenate Strings("Auton File: ", w26) -> (w25:string)
  n135 = call <vilib>:"WPI_DriverStationLCDWrite User Message.vi"("line text"=w25, "line"=WPI_DriverStationLCDLCDLine."User - Line 6", "starting column"=i8 1) -> ()  [unwired: 2 in, 11 out]
